vi "MTM2_logEvent_tcpIpConnected.vi"(8 "error in (no error)":errorcluster, 11 "logevent_tcpIpConnected_Ctl":T1) -> (0 "error out":errorcluster, 2 "function return":i32, 3 "logevent_tcpIpConnected_Ctl out":T1)   [LabVIEW 2018, in "SALLV_MTM2.lvlib"]
doc: "int MTM2_shm_logEvent_tcpIpConnectedLV(MTM2_logevent_tcpIpConnectedLV *logevent_tcpIpConnected_Ctl );"
uses:
  DataTypes/logevent_tcpIpConnected.ctl
  SALLV_MTM2.lvlib
  SALLV_MTM2.so
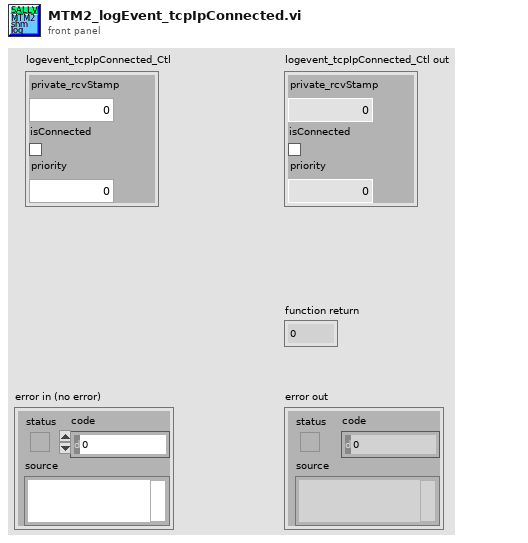
[diagram p1: front panel]
types:
  T1 = typedef "SALLV_MTM2.lvlib/logevent_tcpIpConnected.ctl" = cluster{"private_rcvStamp":dbl, "isConnected":bool, "priority":i32}
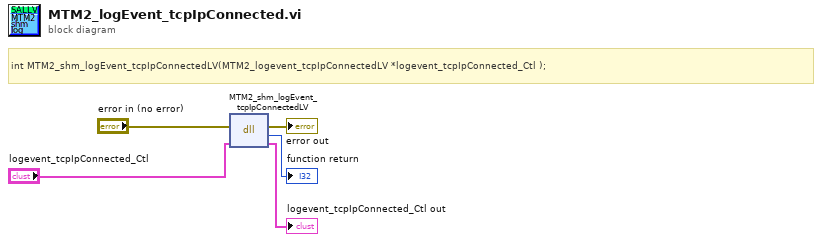
[diagram p0: block diagram]
diagram:
  # "int MTM2_shm_logEvent_tcpIpConnectedLV(MTM2_logevent_tcpIpConnectedLV *logevent_tcpIpConnected_Ctl );"
  n1 = dll-call lib="home/ttsai/Documents/salTestLabViewApi/SALLV_MTM2/SALLV_MTM2.*" fn="MTM2_shm_logEvent_tcpIpConnectedLV"(error in="error in (no error)", "logevent_tcpIpConnected_Ctl"="logevent_tcpIpConnected_Ctl") -> (error out=→"error out":errorcluster, →"function return":i32, "logevent_tcpIpConnected_Ctl"=→"logevent_tcpIpConnected_Ctl out":T1)  [unwired: 2 in, 1 out]
